vi "Z Aux Get Modbus Mpos.vi"(8 "error in (no error)":errorcluster caption="错误输入（无错误）", 9 "pValueList":sgl, 10 "imaxaxises":i32, 11 "handle":u32) -> (0 "error out":errorcluster caption="错误输出", 1 "pValueList out":sgl, 2 "function return":i32, 3 "handle out":u32)   [LabVIEW 2015, in "zauxdll.lvlib"]
doc: "int32 __stdcall ZAux_GetModbusMpos(ZMC_HANDLE handle, int imaxaxises, float *pValueList);"
uses:
  zauxdll.lvlib
  zauxdll.dll
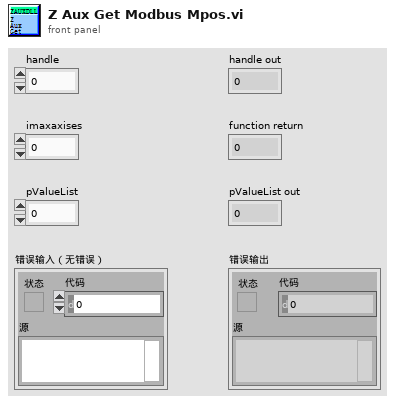
[diagram p1: front panel]
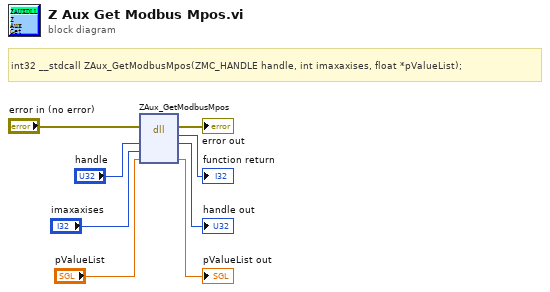
[diagram p0: block diagram]
diagram:
  # "int32 __stdcall ZAux_GetModbusMpos(ZMC_HANDLE handle, int imaxaxises, float *pValueList);"
  n1 = dll-call lib="C:/Users/VIC/Desktop/GOGORO_Oringnal - Panasonic/system/LLB/zmotion/zaux/zauxdll.*" fn="ZAux_GetModbusMpos"(error in="error in (no error)", "handle"="handle", "imaxaxises"="imaxaxises", "pValueList"="pValueList") -> (error out=→"error out":errorcluster, →"function return":i32, "handle"=→"handle out":u32, "pValueList"=→"pValueList out":sgl)  [unwired: 3 in, 1 out]
